vi "rtd measure (fpga).vi"() -> ()   [LabVIEW 2012]
uses:
  <vilib>/rvi/eio/common/nirviEmuTemplateMethod_errors.vi
  <vilib>/eio/EIONode/EIONode.xnode
panel:
  out "Chassis2/Mod3/RTD3":fxp<+/-,24,10>
  out "Chassis2/Mod3/RTD2":fxp<+/-,24,10>
  out "Chassis2/Mod3/RTD1":fxp<+/-,24,10>
  out "Chassis2/Mod3/RTD0":fxp<+/-,24,10>
  in  "Count(Ticks)":u32=8000000
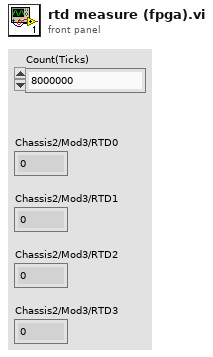
[diagram p1: front panel]
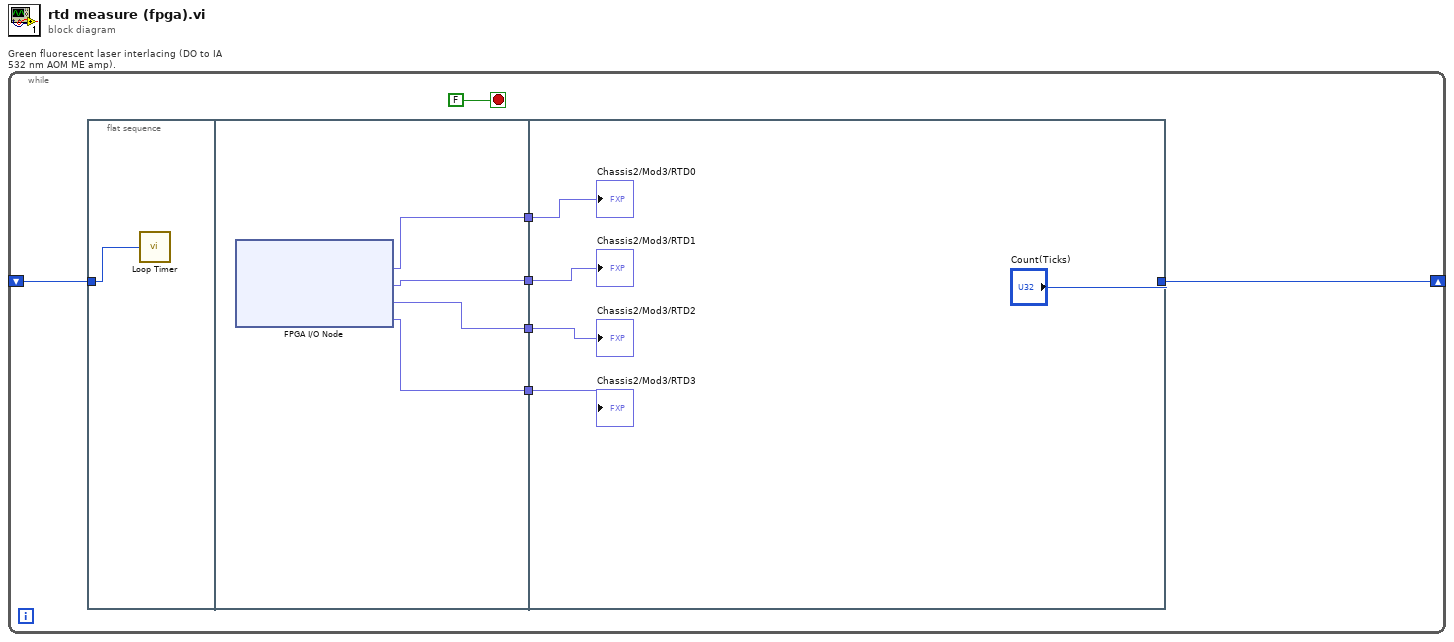
[diagram p0: block diagram]
diagram:
  n1 = while "Green fluorescent laser interlacing (DO to IA 532 nm AOM ME amp)." {
    shift-right: [w5] -> _
    shift-left: _ -> [w6]
    stop <- FALSE stop-if-true
    n2 = flat-sequence {
      tunnel: w6 -> [w8]
      tunnel: [w12] -> w4
      tunnel: [w11] -> w3
      tunnel: [w10] -> w2
      tunnel: [w9] -> w1
      tunnel: ["Count(Ticks)"] -> w5
      tunnel: w4 -> [w16]
      tunnel: w3 -> [w15]
      tunnel: w2 -> [w14]
      tunnel: w1 -> [w13]
      frame #0 {
        n3 = call "Loop Timer"("Count(Ticks)"=w8) -> ()  [unwired: 1 out]
      }
      frame #1 {
        n4 = xnode "FPGA I/O Node"() -> ("Chassis2/Mod3/RTD0"=w12:fxp<+/-,24,10>, "Chassis2/Mod3/RTD1"=w11:fxp<+/-,24,10>, "Chassis2/Mod3/RTD2"=w10:fxp<+/-,24,10>, "Chassis2/Mod3/RTD3"=w9:fxp<+/-,24,10>)  [unwired: 4 in, 4 out]
      }
      frame #2 {
        "Chassis2/Mod3/RTD0" <- w16
        "Chassis2/Mod3/RTD1" <- w15
        "Chassis2/Mod3/RTD2" <- w14
        "Chassis2/Mod3/RTD3" <- w13
      }
    }
  }
